vi "Get Client Operation.vi"(8 "error in (no error)":errorcluster, 11 "Request in":refnum<class "Request.lvclass">) -> (0 "error out":errorcluster, 2 "Client Operation":T1, 3 "Request out":refnum<class "Request.lvclass">)   [LabVIEW 2022 SP3, in "obs-websocket-lv.lvlib" / "Request.lvclass"]
uses:
  Request.lvclass
  Client Operation.ctl
  Request.lvclass/Request.ctl
  obs-websocket-lv.lvlib
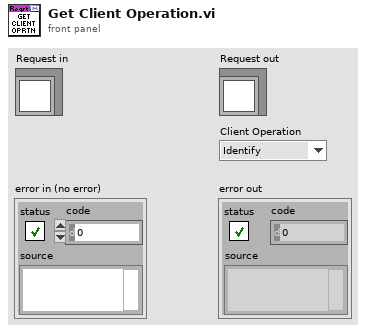
[diagram p1: front panel]
types:
  T1 = typedef "obs-websocket-lv.lvlib/Client Operation.ctl" = enum16{"Identify", "Reidentify", "Request", "RequestBatch"}
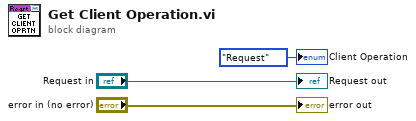
[diagram p0: block diagram]
diagram:
  "error out" <- "error in (no error)"
  "Request out" <- "Request in"
  "Client Operation" <- Client_Operation."Request" ("Client Operation")
